vi "ConnectToDatabase.vi"(8 "error in":errorcluster) -> (0 "error out":errorcluster, 3 "Database ref":refnum<k24>)   [LabVIEW 2015]
uses:
  C:/Users/Bartek/Desktop/NORDIC/NORDIC LabVIEW GUI/DLLs/NordicDatabaseDLL.dll
  DLLs/NordicDatabaseDLL.dll
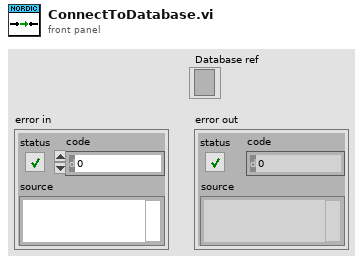
[diagram p1: front panel]
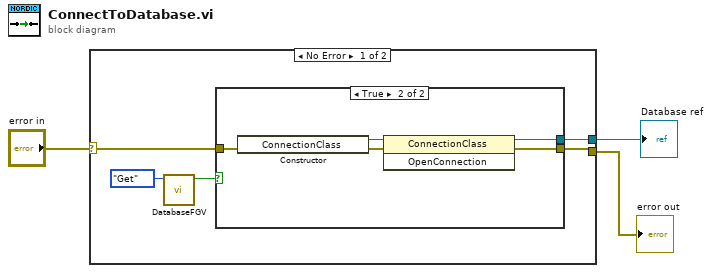
[diagram p0: block diagram]
diagram:
  n1 = case shown="No Error" "error in" {
    selector: "error in" -> [w7 w15]
    tunnel: [w8 _] -> w3
    tunnel: [w6 w15] -> w1
    frame No Error {
      n2 = call "DatabaseFGV.vi"("State"=enum16{"Get", "Set"}."Get") -> ("Active?"=w4:bool)  [unwired: 10 in]
      n3 = case shown="True" w4 {
        tunnel: [_ w14] -> w8
        tunnel: w7 -> [w9 w13]
        tunnel: [w9 w12] -> w6
        frame False {
        }
        frame True {
          n4 = constructor class="ConnectionClass"(error in=w13) -> (reference out=w11:refnum<k24>, error out=w10:errorcluster)  [unwired: 2 in, 1 out]
          n5 = invoke class="ConnectionClass" method="OpenConnection"(reference=w11, error in=w10) -> (reference out=w14:refnum<k24>, error out=w12:errorcluster)  [unwired: 1 in, 1 out]
        }
      }
    }
    frame Error {
    }
  }
  "Database ref" <- w3
  "error out" <- w1
